vi "NicmosGetData.vi"(9 "error in (no error)":errorcluster caption="error out (no error)") -> (2 "DATA":T1, 6 "error out":errorcluster)   [LabVIEW 2009]
uses:
  Controls/NICMOS.DATA.ctl
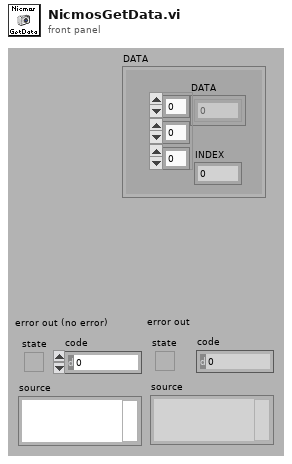
[diagram p1: front panel]
types:
  T1 = typedef "NICMOS.DATA.ctl" = cluster{"DATA":i32[][][], "INDEX":i32}
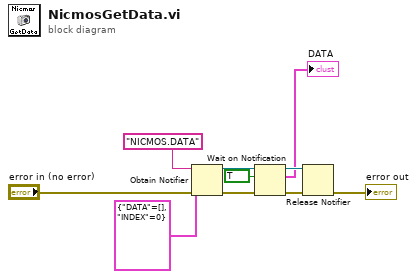
[diagram p0: block diagram]
diagram:
  n1 = Obtain Notifier(name (unnamed)="NICMOS.DATA" ("nom (aucun)"), notification data type=T1 {"DATA"=[], "INDEX"=0}, error in (no error)="error in (no error)") -> (notifier out=w5:refnum<notifier>, error out=w9:errorcluster)  [unwired: 1 in, 1 out]
  n2 = Wait on Notification(notifier=w5, ignore previous (F)=TRUE, error in (no error)=w9) -> (notifier out=w4:refnum<notifier>, notification=→"DATA":T1, error out=w8:errorcluster)  [unwired: 1 in, 1 out]
  n3 = Release Notifier(notifier=w4, error in (no error)=w8) -> (error out=→"error out":errorcluster)  [unwired: 1 in, 2 out]
